vi "Read Null.vi"(0 "FlexChannel":T1) -> ()   [LabVIEW 2020, in "Flex.lvlib"]
doc: "Terminates a Channel Wire without any transactions. This can be useful to terminate a Channel Wire branch on an existing API that isn't needed in an application."
uses:
  Flex.lvlib
  ChannelOp.ctl
  Element.ctl
  ))Channel.ctl
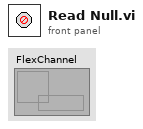
[diagram p1: front panel]
types:
  T1 = typedef "Flex.lvlib/))Channel.ctl" = refnum<queue>
  T2 = typedef "Flex.lvlib/ChannelOp.ctl" = enum16{"Get Refs", "Init", "Close", "Probe", "New Queue", "Remove Queue", "New Event"}
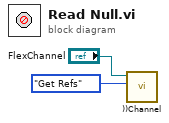
[diagram p0: block diagram]
diagram:
  n1 = call "))Channel.vi"("channelOp"=ChannelOp."Get Refs", "channel in"="FlexChannel") -> ()  [unwired: 5 in, 5 out]
